vi "Read Piece.vi"(11 "Move in":refnum<class "Move.lvclass">) -> (2 "Chesslib.lvlib:Piece.lvclass":refnum<class "Piece.lvclass">, 3 "Move out":refnum<class "Move.lvclass">)   [LabVIEW 2015, in "Chesslib.lvlib" / "Move.lvclass"]
uses:
  Move.lvclass
  Pieces/Piece/Piece.lvclass
  Move.lvclass/Move.ctl
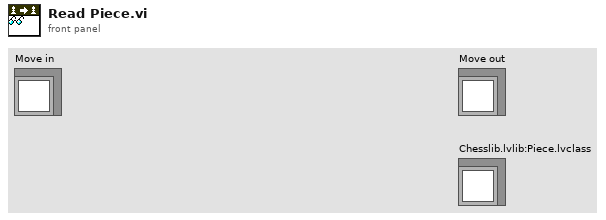
[diagram p1: front panel]
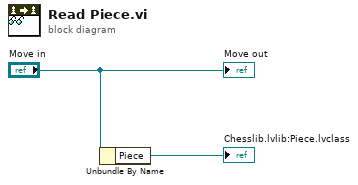
[diagram p0: block diagram]
diagram:
  n1 = Unbundle By Name("Move in") -> ("Piece"=→"Chesslib.lvlib:Piece.lvclass":refnum<class "Piece.lvclass">)
  "Move out" <- "Move in"
